vi "Print.vi"(6 "Byte Count (1024)":u32=1024, 7 "Timeout (2000 ms)":u32=2000, 8 "error in (no error)":errorcluster, 9 "Input":string, 11 "VISA resource name":refnum<visa-resource-name>) -> (0 "error out":errorcluster, 1 "Output":string, 2 "Return Count":u32, 3 "VISA resource name out":refnum<visa-resource-name>, 4 "Command String":string)   [LabVIEW 2018, in "Keithley 2600 Series.lvlib"]
doc: "This VI instructs the instrument to print the contents of the test script variable or value named by Input, to the instrument's output data queue.\n\n<b>Note:</b> Floating point values will be printed with the number of digits specified by format.asciiprecision.\n\n<b>Functions and Attributes Used</b>\nprint()"
uses:
  Keithley 2600 Series.lvlib
  Private/GlobalVariables.vi
panel:
  # "(c) 2008 Keithley Instruments, Inc.  ALL RIGHTS RESERVED."
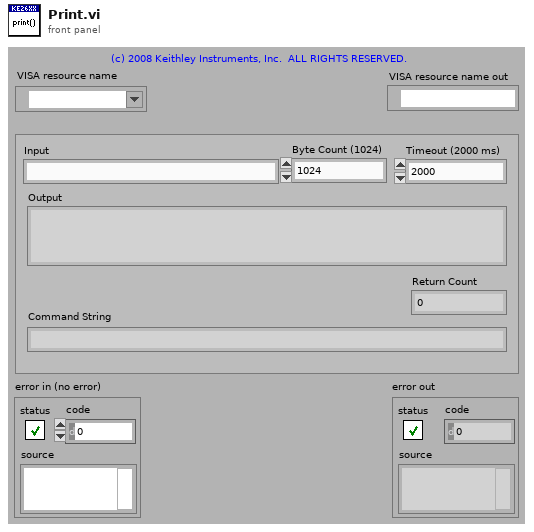
[diagram p1: front panel]
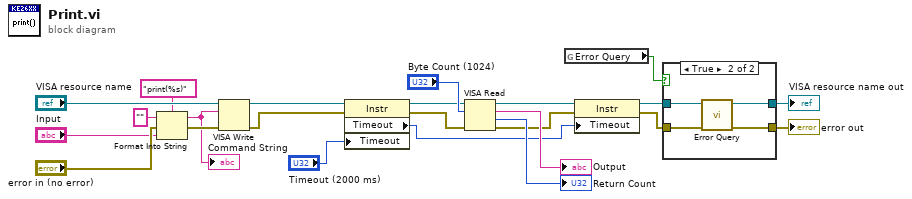
[diagram p0: block diagram]
diagram:
  n1 = Format Into String(format string="print(%s)", initial string="", error in="error in (no error)", "Input") -> (resulting string=w16:string, error out=w20:errorcluster)
  "Command String" <- w16
  n2 = VISA Write(VISA resource name="VISA resource name", write buffer=w16, error in (no error)=w20) -> (VISA resource name out=w10:refnum<visa-resource-name>, error out=w9:errorcluster)  [unwired: 1 out]
  n3 = property class="Instr"(reference=w10, error in=w9, "Timeout"="Timeout (2000 ms)") -> (reference out=w8:refnum<visa-resource-name>, error out=w7:errorcluster, "Timeout"=w4:u32)
  n4 = VISA Read(VISA resource name=w8, byte count="Byte Count (1024)", error in (no error)=w7) -> (VISA resource name out=w6:refnum<visa-resource-name>, read buffer=→"Output":string, return count=→"Return Count":u32, error out=w5:errorcluster)
  n5 = global read "GlobalVariables.vi" "Error Query"() -> (w15:bool)
  n6 = property class="Instr"(reference=w6, error in=w5, "Timeout"=w4) -> (reference out=w2:refnum<visa-resource-name>, error out=w3:errorcluster)
  n7 = case shown="True" w15 {
    tunnel: w2 -> [w25 w29]
    tunnel: w3 -> [w24 w28]
    tunnel: [w25 w27] -> w14
    tunnel: [w24 w26] -> w23
    frame False {
    }
    frame True {
      n8 = call "Error Query.vi"("error in (no error)"=w28, "VISA resource name"=w29) -> ("error out"=w26:errorcluster, "VISA resource name out"=w27:refnum<visa-resource-name>)  [unwired: 8 out]
    }
  }
  "error out" <- w23
  "VISA resource name out" <- w14
